vi "Obtain Session (Port).vi"(0 "Remote Listener  ID ()":string, 1 "port number (3363)":u16=3363, 2 "remote machine name (Current App:\"\")":string(combo), 11 "error in (no error)":errorcluster) -> (4 "Session Handle":T1, 8 "created new?":bool, 15 "error out":errorcluster)   [LabVIEW 2012, in "REx.lvlib" / "Remote Connection Session.lvclass"]
doc: "This function initializes the measurement\n\nPass the function a name to obtain an active measurement handle"
uses:
  Remote Connection Session.lvclass
  Typedefs/Session Handle.ctl
  Remote Connection Session.lvclass/Remote Connection Session.ctl
  Utilities/initialize Session Data.vi
  <userlib>/_Session Fwk/Session - Root.lvclass
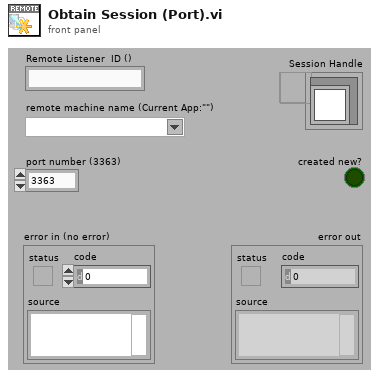
[diagram p1: front panel]
types:
  T1 = typedef "REx.lvlib/Remote Connection Session.lvclass/Session Handle.ctl" = refnum<data-value>
  T2 = typedef "Session - Root.lvclass/Session Handle.ctl" = refnum<data-value>
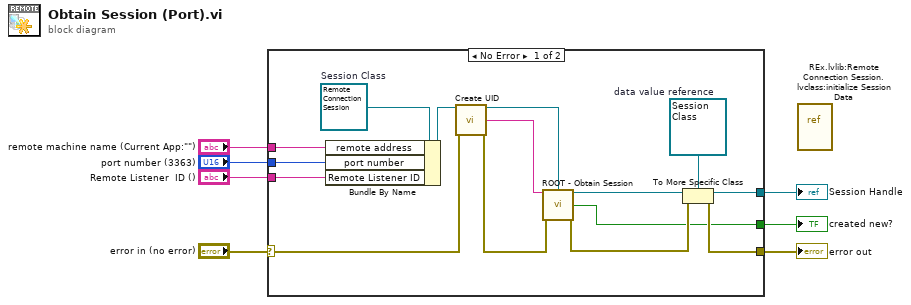
[diagram p0: block diagram]
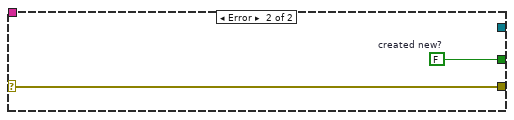
[diagram p2: hidden frame]
diagram:
  n1 = case shown="No Error" "error in (no error)" {
    selector: "error in (no error)" -> [w12 w24]
    tunnel: [w20 w24] -> w6
    tunnel: [w22 _] -> w4
    tunnel: "Remote Listener  ID ()" -> [w14 _]
    tunnel: "port number (3363)" -> [w16 _]
    tunnel: "remote machine name (Current App:\"\")" -> [w15 _]
    tunnel: [w8 w23] -> w1
    frame No Error {
      w17 = refnum<data-value> refnum  # data value reference
      w18 = refnum<class "Remote Connection Session.lvclass"> refnum  # Session Class
      n2 = Bundle By Name(cluster=w18, "remote address"=w15, "port number"=w16, "Remote Listener ID"=w14) -> (w10:refnum<class "Remote Connection Session.lvclass">)
      n3 = call "Create UID.vi"("Remote Connection Session in"=w10, "error in (no error)"=w12) -> ("Remote Connection Session out"=w9:refnum<class "Remote Connection Session.lvclass">, "Session UID"=w13:string, "error out"=w11:errorcluster)  [unwired: 11 in]
      n4 = call <userlib>:"ROOT - Obtain Session.vi"("Session Name ()"=w13, "OBJ - Session"=w9, "error in (no error)"=w11) -> ("Session Handle"=w19:T2, "created new?"=w8:bool, "error out"=w21:errorcluster)  [unwired: 10 in]
      n5 = To More Specific Class(target class=w17, reference=w19, error in=w21) -> (specific class reference=w22:refnum<data-value>, error out=w20:errorcluster)
    }
    frame Error {
      w23 = FALSE  # created new?
    }
  }
  "error out" <- w6
  "Session Handle" <- w4
  "created new?" <- w1
  n6 = vi-ref "REx.lvlib:Remote Connection Session.lvclass:initialize Session Data.vi"() -> ()  [unwired: 1 out]
